vi "Mean Stimulus Coefficients.vi"(1 "Coefficients in":T1[](array[typedef]) {"Freq" format="%#.2f"; "Offset" format="%.3f"; "Gain" format="%.2f"; "Phase" format="%.1f"}) -> (0 "Mean Coefficients out":T1 {"Freq" format="%#.2f"; "Offset" format="%.3f"; "Gain" format="%.2f"; "Phase" format="%.1f"})   [LabVIEW 2013, in "Sinusoidal Fit.lvclass"]
uses:
  Sinusoidal Fit.lvclass
  gain and phase/Typedef - Sinusoidal Fit Coefficients.ctl
  comm/nan operations/nan operations.lvlib
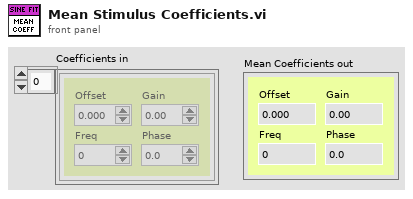
[diagram p1: front panel]
types:
  T1 = typedef "Typedef - Sinusoidal Fit Coefficients.ctl" = cluster{"Offset":dbl, "Gain":dbl, "Phase":dbl, "Freq":dbl}
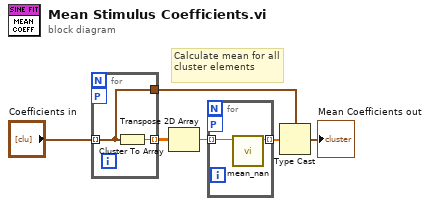
[diagram p0: block diagram]
diagram:
  # "Calculate mean for all cluster elements"
  n1 = for {
    workers-P: _ -> [_]
    tunnel: "Coefficients in" -> [w7] mode=indexing
    tunnel: [w8] -> w4 mode=indexing
    tunnel: [w7] -> w2
    n2 = Cluster To Array(cluster=w7) -> (array=w8:dbl[])
  }
  n3 = Transpose 2D Array(2D array=w4) -> (transposed array=w3:dbl[][])
  n4 = for {
    tunnel: w3 -> [w10] mode=indexing
    tunnel: [w9] -> w6 mode=indexing
    workers-P: _ -> [_]
    n5 = call "mean_nan.vi"("Array"=w10) -> ("Mean"=w9:dbl)  [unwired: 10 in]
  }
  n6 = Type Cast(type=w2, x=w6) -> (*(type *) &x=→"Mean Coefficients out":T1)
